vi "Add BC to RT Message.vi"(4 "create timestamp channel":bool, 6 "parameters":T2(array[cluster]), 7 "number of words":u16=1, 8 "error in":errorcluster, 9 "remote terminals":cluster{"Rx":T3, "Tx":T3}, 10 "name":string, 11 "port in":T5 format="%.0x") -> (0 "error out":errorcluster, 3 "port out":T5 format="%.0x")   [LabVIEW 2020, in "Ballard MIL-STD-1553 Scripting.lvlib"]
uses:
  Ballard MIL-STD-1553 Scripting.lvlib
  <vilib>/NI VeriStand/Custom Device API/Custom Device Item Ref.ctl
  Shared/Terminal Endpoint.ctl
  Shared/Address.ctl
  Shared/Parameter Definition.ctl
  Shared/Direction.ctl
  <vilib>/NI VeriStand/Custom Device API/Custom Device API.lvlib
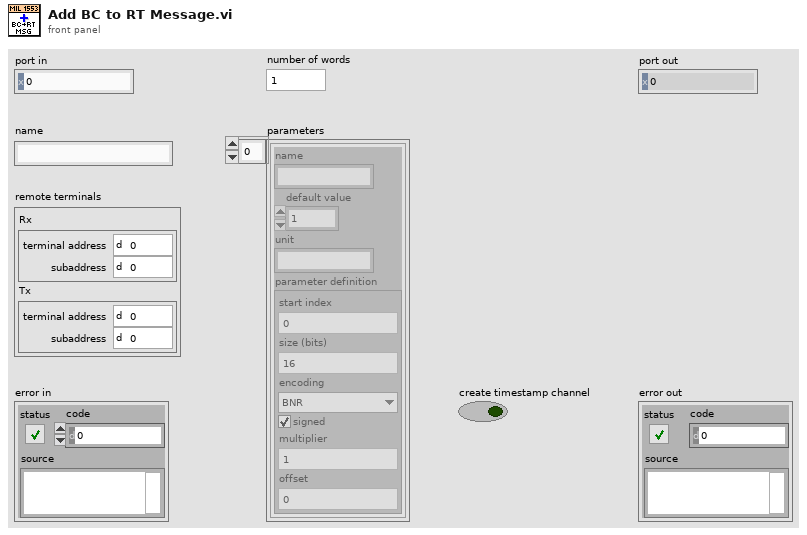
[diagram p1: front panel]
types:
  T1 = typedef "Parameter Definition.ctl" = cluster{"start index":i32, "size (bits)":i32, "encoding":enum16{"BNR", "BCD", "Discrete"}, "signed":bool, "multiplier":dbl, "offset":dbl}
  T2 = cluster{"name":string, "default value":dbl, "unit":string, "parameter definition":T1}[]
  T3 = typedef "Terminal Endpoint.ctl" = cluster{"terminal address":T4, "subaddress":T4}
  T4 = typedef "Address.ctl" = u16
  T5 = typedef "Custom Device API.lvlib/Custom Device Item Ref.ctl" = u64
  T6 = typedef "Direction.ctl" = enum16{"Rx", "Tx"}
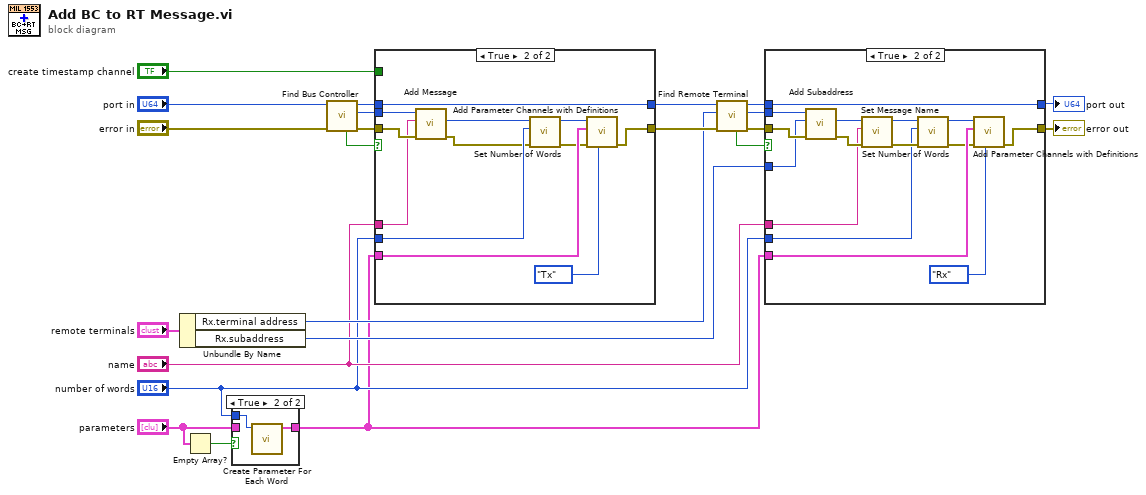
[diagram p0: block diagram]
diagram:
  n1 = Unbundle By Name("remote terminals") -> ("Rx.terminal address"=w8:T4, "Rx.subaddress"=w6:T4)
  n2 = Empty Array?(array="parameters") -> (empty?=w4:bool)
  n3 = case shown="True" w4 {
    tunnel: "number of words" -> [_ w26]
    tunnel: "parameters" -> [w24 _]
    tunnel: [w24 w25] -> w1
    frame False {
    }
    frame True {
      n4 = call "Create Parameter For Each Word.vi"("number of words"=w26) -> ("parameters"=w25:T2)  [unwired: 9 in, 1 out]
    }
  }
  n5 = call "Find Bus Controller.vi"("error in"="error in", "port in"="port in") -> ("error out"=w18:errorcluster, "bus controller"=w19:T5, "port out"=w20:T5, "found?"=w21:bool)  [unwired: 6 in]
  n6 = case shown="True" w21 {
    tunnel: w20 -> [w28 w39]
    tunnel: w19 -> [_ w38]
    tunnel: w18 -> [w27 w40]
    tunnel: [w27 w36] -> w12
    tunnel: [w28 w39] -> w11
    tunnel: "create timestamp channel" -> [_ _]
    tunnel: "number of words" -> [_ w37]
    tunnel: w1 -> [_ w35]
    tunnel: "name" -> [_ w29]
    frame False {
    }
    frame True {
      n7 = call "Add Message.vi"("error in"=w40, "message name"=w29, "bus controller in"=w38) -> ("error out"=w32:errorcluster, "message"=w33:T5)  [unwired: 6 in, 1 out]
      n8 = call "Set Number of Words.vi"("error in"=w32, "number of words"=w37, "message in"=w33) -> ("error out"=w30:errorcluster, "message out"=w31:T5)  [unwired: 7 in]
      n9 = call "Add Parameter Channels with Definitions.vi"("direction"=Direction."Tx", "error in"=w30, "parameters"=w35, "message in"=w31) -> ("error out"=w36:errorcluster)  [unwired: 6 in, 1 out]
    }
  }
  n10 = call "Find Remote Terminal.vi"("error in"=w12, "terminal address"=w8, "port in"=w11) -> ("error out"=w16:errorcluster, "remote terminal"=w15:T5, "port out"=w14:T5, "found?"=w13:bool)  [unwired: 5 in]
  n11 = case shown="True" w13 {
    tunnel: w14 -> [w42 w56]
    tunnel: w15 -> [_ w55]
    tunnel: w16 -> [w41 w57]
    tunnel: [w41 w51] -> w9
    tunnel: [w42 w56] -> w10
    tunnel: w6 -> [_ w54]
    tunnel: "number of words" -> [_ w43]
    tunnel: w1 -> [_ w53]
    tunnel: "name" -> [_ w44]
    frame False {
    }
    frame True {
      n12 = call "Add Subaddress.vi"("error in"=w57, "subaddress"=w54, "remote terminal in"=w55) -> ("error out"=w49:errorcluster, "subaddress ref"=w50:T5)  [unwired: 6 in, 1 out]
      n13 = call "Set Message Name.vi"("error in"=w49, "message name"=w44, "message in"=w50) -> ("error out"=w47:errorcluster, "message out"=w48:T5)  [unwired: 7 in]
      n14 = call "Set Number of Words.vi"("error in"=w47, "number of words"=w43, "message in"=w48) -> ("error out"=w45:errorcluster, "message out"=w46:T5)  [unwired: 7 in]
      n15 = call "Add Parameter Channels with Definitions.vi"("direction"=Direction."Rx", "error in"=w45, "parameters"=w53, "message in"=w46) -> ("error out"=w51:errorcluster)  [unwired: 6 in, 1 out]
    }
  }
  "error out" <- w9
  "port out" <- w10
